vi "ROM Data.vi"(2 "Value from LPCA":string, 3 "Command":enum16{"Init", "Get Index", "Analyze"}(ring)) -> (0 "ROM Data":string, 1 "Index":i32)   [LabVIEW 2017]
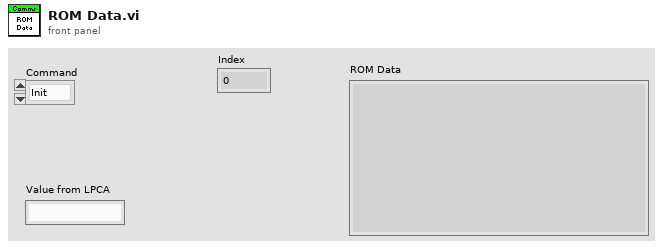
[diagram p1: front panel]
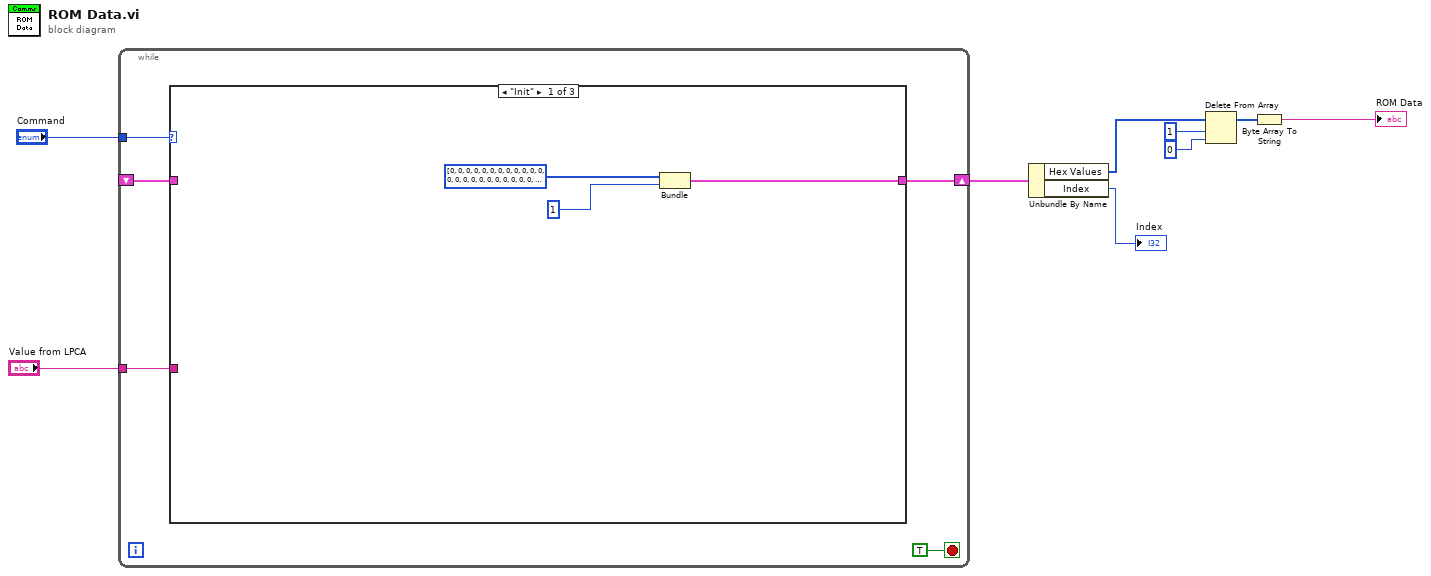
[diagram p0: block diagram]
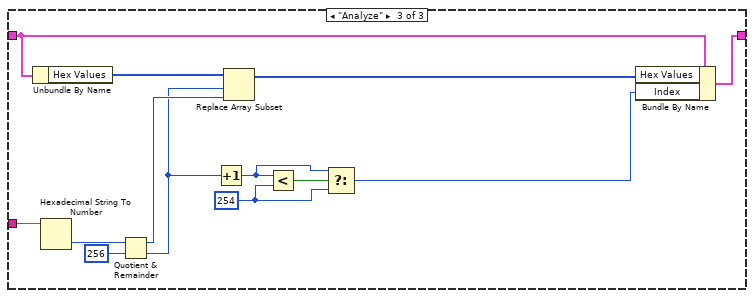
[diagram p3: hidden frame]
diagram:
  n1 = while {
    tunnel: "Command" -> [w14]
    tunnel: "Value from LPCA" -> [w13]
    shift-right: [w12] -> w7
    shift-left: _ -> [w11]
    stop <- TRUE stop-if-true
    n2 = case shown="\"Init\"" w14 {
      tunnel: w13 -> [_ _ w30]
      tunnel: [w15 w18 w31] -> w12
      tunnel: w11 -> [_ w18 w27]
      frame "Init" {
        n3 = Bundle("Hex Values"=u8[] [0, 0, 0, 0, 0, 0, 0, 0, 0, 0, 0, 0, 0, 0, 0, 0, 0, 0, 0, 0, 0, 0, 0, 0, 0, 0, 0, 0, 0, 0, 0, 0, 0, 0, 0, 0, 0, 0, 0, 0, 0, 0, 0, 0, 0, 0, 0, 0, 0, 0, 0, 0, 0, 0, 0, 0, 0, 0, 0, 0, 0, 0, 0, 0, 0, 0, 0, 0, 0, 0, 0, 0, 0, 0, 0, 0, 0, 0, 0, 0, 0, 0, 0, 0, 0, 0, 0, 0, 0, 0, 0, 0, 0, 0, 0, 0, 0, 0, 0, 0, 0, 0, 0, 0, 0, 0, 0, 0, 0, 0, 0, 0, 0, 0, 0, 0, 0, 0, 0, 0, 0, 0, 0, 0, 0, 0, 0, 0, 0, 0, 0, 0, 0, 0, 0, 0, 0, 0, 0, 0, 0, 0, 0, 0, 0, 0, 0, 0, 0, 0, 0, 0, 0, 0, 0, 0, 0, 0, 0, 0, 0, 0, 0, 0, 0, 0, 0, 0, 0, 0, 0, 0, 0, 0, 0, 0, 0, 0, 0, 0, 0, 0, 0, 0, 0, 0, 0, 0, 0, 0, 0, 0, 0, 0, 0, 0, 0, 0, 0, 0, 0, 0, 0, 0, 0, 0, 0, 0, 0, 0, 0, 0, 0, 0, 0, 0, 0, 0, 0, 0, 0, 0, 0, 0, 0, 0, 0, 0, 0, 0, 0, 0, 0, 0, 0, 0, 0, 0, 0, 0, 0, 0, 0, 0, 0, 0, 0, 0, 0, 0, 0, 0, 0, 0, 0, 0], "Index"=1) -> (w15:cluster{"Hex Values":u8[], "Index":i32})  [unwired: 1 in]
      }
      frame "Get Index" {
      }
      frame "Analyze" {
        w19 = u32 254 ("y")
        n4 = Unbundle By Name(w27) -> ("Hex Values"=w26:u8[])
        n5 = Hexadecimal String To Number(string=w30) -> (number=w29:u32)  [unwired: 2 in, 1 out]
        n6 = Quotient & Remainder(x=w29, y=u32 256) -> (x-y*floor(x/y)=w25:u32, floor(x/y)=w23:u32)
        n7 = Increment(x=w23) -> (x+1=w21:u32)
        n8 = Replace Array Subset(array=w26, new element=w25, index=w23) -> (w24:u8[])
        n9 = Less?(x=w21, y=w19) -> (x < y?=w22:bool)
        n10 = Select(t=w21, s=w22, f=w19) -> (s? t:f=w20:u32)
        n11 = Bundle By Name(cluster=w27, "Hex Values"=w24, "Index"=w20) -> (w31:cluster{"Hex Values":u8[], "Index":i32})
      }
    }
  }
  n12 = Unbundle By Name(w7) -> ("Hex Values"=w5:u8[], "Index"=→"Index":i32)
  n13 = Delete From Array(array=w5, length=1, index=0) -> (array with subset deleted=w4:u8[])  [unwired: 1 out]
  n14 = Byte Array To String(unsigned byte array=w4) -> (string=→"ROM Data":string)
